vi "Open DB.vi"(8 "error in (no error)":errorcluster, 11 "LV-ORM in":refnum<class "LV-ORM.lvclass">) -> (0 "error out":errorcluster, 3 "LV-ORM out":refnum<class "LV-ORM.lvclass">)   [LabVIEW 2018, in "LV-ORM.lvclass"]
uses:
  LV-ORM.lvclass
  LV-ORM.lvclass/LV-ORM.ctl
  <vilib>/addons/database/Connection.llb/DB Tools Open Connec (Path).vi
  <vilib>/addons/database/NI_Database_API.lvlib
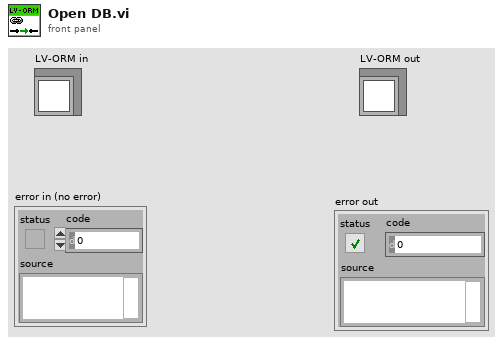
[diagram p1: front panel]
types:
  T1 = typedef "NI_Database_API.lvlib/Conn ObjectReference.ctl" = refnum<k1>
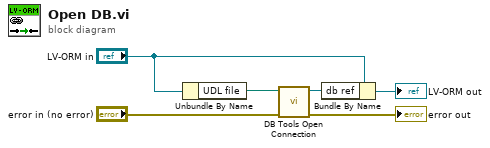
[diagram p0: block diagram]
diagram:
  n1 = Unbundle By Name("LV-ORM in") -> ("UDL file"=w1:path)
  n2 = call-poly <vilib>:"DB Tools Open Connection.vi"("error in (no error)"="error in (no error)", "connection information"=w1) -> ("error out"=→"error out":errorcluster, "connection reference"=w4:T1)  [unwired: 6 in]
  n3 = Bundle By Name(cluster="LV-ORM in", "db ref"=w4) -> (→"LV-ORM out":refnum<class "LV-ORM.lvclass">)
